vi "档位判断.vi"(1 "数值":dbl) -> (0 "数组":bool[](array[boolean]))   [LabVIEW 8.6]
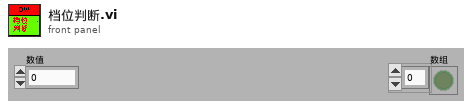
[diagram p1: front panel]
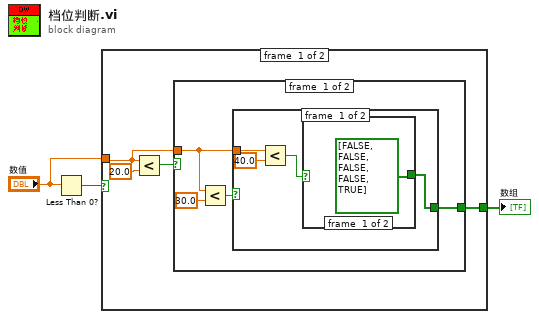
[diagram p0: block diagram]
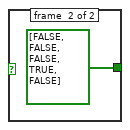
[diagram p2: hidden frame]
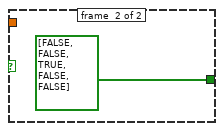
[diagram p3: hidden frame]
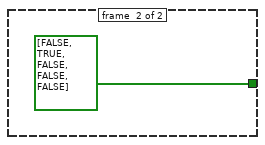
[diagram p4: hidden frame]
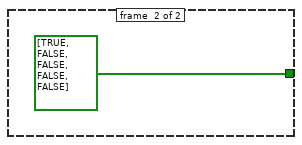
[diagram p5: hidden frame]
diagram:
  n1 = Less Than 0?(x="数值") -> (x < 0?=w3:bool)
  n2 = case shown="假" w3 {
    tunnel: [w5 bool[] [TRUE, FALSE, FALSE, FALSE, FALSE]] -> w1
    tunnel: "数值" -> [w4 _]
    frame #0 {
      n3 = Less?(x=w4, y=20.0) -> (x < y?=w6:bool)
      n4 = case shown="假" w6 {
        tunnel: [w9 bool[] [FALSE, TRUE, FALSE, FALSE, FALSE]] -> w5
        tunnel: w4 -> [w8 _]
        frame #0 {
          n5 = Less?(x=w8, y=30.0) -> (x < y?=w10:bool)
          n6 = case shown="假" w10 {
            tunnel: [w12 bool[] [FALSE, FALSE, TRUE, FALSE, FALSE]] -> w9
            tunnel: w8 -> [w15 _]
            frame #0 {
              n7 = Less?(x=w15, y=40.0) -> (x < y?=w13:bool)
              n8 = case shown="假" w13 {
                tunnel: [bool[] [FALSE, FALSE, FALSE, FALSE, TRUE] bool[] [FALSE, FALSE, FALSE, TRUE, FALSE]] -> w12
                frame #0 {
                }
                frame #1 {
                }
              }
            }
            frame #1 {
            }
          }
        }
        frame #1 {
        }
      }
    }
    frame #1 {
    }
  }
  "数组" <- w1
